vi "Create UI.vi"(8 "error in (no error)":errorcluster, 10 "Instrument in":refnum<class "Instrument.lvclass">, 11 "Instrument.Cryostation UI in":refnum<class "Instrument.Cryostation UI.lvclass">) -> (0 "error out":errorcluster, 3 "Instrument.Cryostation UI out":refnum<class "Instrument.Cryostation UI.lvclass">)   [LabVIEW 2016, in "Instrument.Cryostation UI.lvclass"]
uses:
  Instrument.Cryostation UI.lvclass
  C:/Program Files (x86)/National Instruments/LabVIEW 2016/vi.lib/JKI/JKI SMO/SMO/SMO.lvclass
  <userlib>/LevyLab/Levylab Instruments/SMOs/Instrument/Instrument.lvclass
  Instrument.Cryostation UI.lvclass/Instrument.Cryostation UI.ctl
  <vilib>/JKI/JKI SMO/SMO/SMO.lvclass
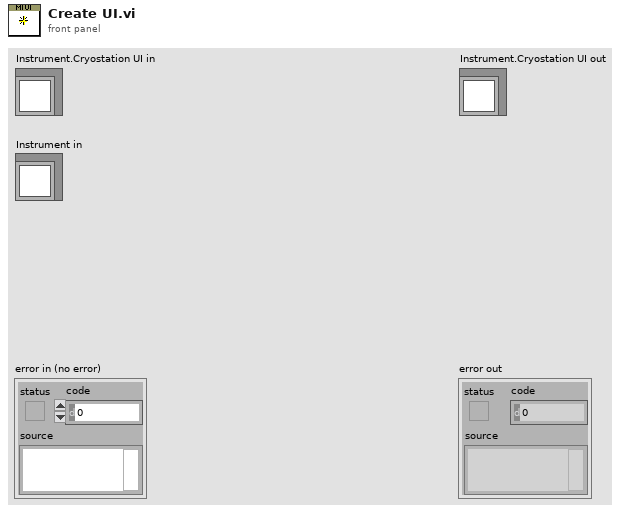
[diagram p1: front panel]
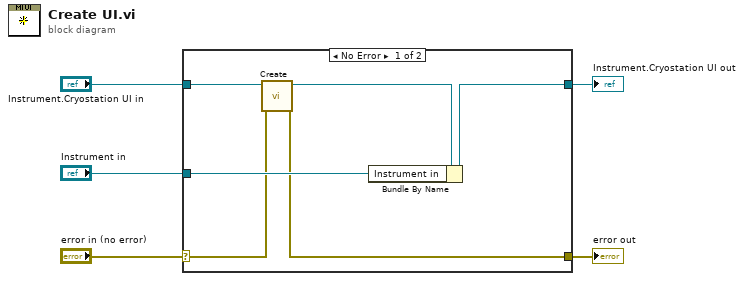
[diagram p0: block diagram]
diagram:
  n1 = case shown="No Error" "error in (no error)" {
    selector: "error in (no error)" -> [w8 w12]
    tunnel: [w7 w12] -> w4
    tunnel: [w6 w13] -> w2
    tunnel: "Instrument.Cryostation UI in" -> [w10 w13]
    tunnel: "Instrument in" -> [w11 _]
    frame No Error {
      n2 = call <vilib>:"Create.vi"("error in (no error)"=w8, "SMO"=w10) -> ("error out"=w7:errorcluster, "SMO out"=w9:refnum<class "Instrument.Cryostation UI.lvclass">)  [unwired: 7 in, 1 out]
      n3 = Bundle By Name(cluster=w9, "Instrument in"=w11) -> (w6:refnum<class "Instrument.Cryostation UI.lvclass">)
    }
    frame Error {
    }
  }
  "error out" <- w4
  "Instrument.Cryostation UI out" <- w2
